vi "Арифметика1.vi"(2 "C":bool, 3 "B":bool, 4 "A":bool) -> (0 "C":bool, 1 "SUM":bool)   [LabVIEW 2017]
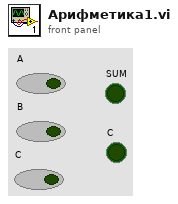
[diagram p1: front panel]
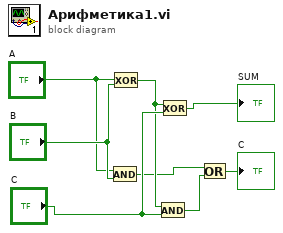
[diagram p0: block diagram]
diagram:
  n1 = And(x="A", y="B") -> (x .and. y?=w1:bool)
  n2 = Exclusive Or(1:"B", 2:"A") -> (0:w4:bool)
  n3 = And(x=w4, y="C") -> (x .and. y?=w2:bool)
  n4 = Exclusive Or(1:"C", 2:w4) -> (0:→"SUM":bool)
  n5 = Or(x=w1, y=w2) -> (x .or. y?=→"C":bool)
